vi "ts_tree_set_result.vi"(4 "results.data":string, 6 "results.txt":string, 8 "error in (no error)":errorcluster, 9 "ts.status":bool, 10 "ts.data":T1, 11 "Tree.in":refnum<vi>) -> (0 "error out":errorcluster, 3 "Tree.out":refnum<vi>)   [LabVIEW 2015]
doc: "sets the test step results for a active/parent tag"
uses:
  ts-data.ctl
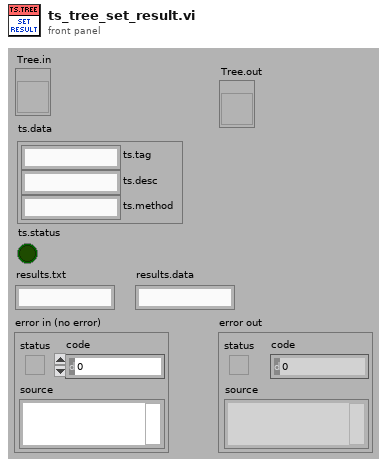
[diagram p1: front panel]
types:
  T1 = typedef "ts-data.ctl" = cluster{"ts.tag":string, "ts.desc":string, "ts.method":string}
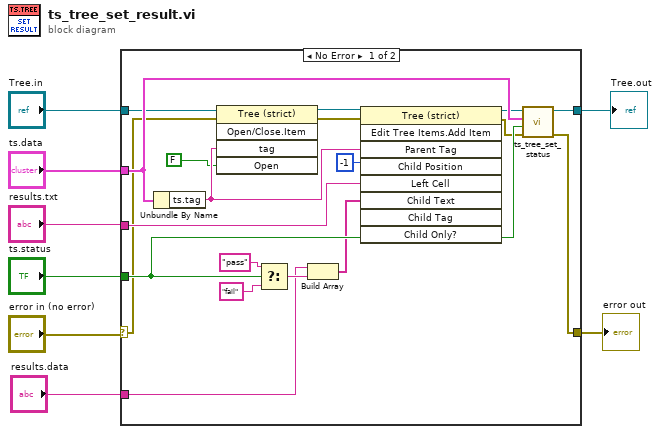
[diagram p0: block diagram]
diagram:
  n1 = case shown="No Error" "error in (no error)" {
    selector: "error in (no error)" -> [w11 w28]
    tunnel: "Tree.in" -> [w14 w29]
    tunnel: [w26 w29] -> w6
    tunnel: [w25 w28] -> w5
    tunnel: "ts.status" -> [w22 _]
    tunnel: "results.txt" -> [w24 _]
    tunnel: "ts.data" -> [w23 _]
    tunnel: "results.data" -> [w18 _]
    frame No Error {
      n2 = Unbundle By Name(w23) -> ("ts.tag"=w10:string)
      n3 = invoke class="Tree (strict)" method="Open/Close.Item"(reference=w14, error in=w11, "tag"=w10, "Open"=FALSE ("Open?")) -> (reference out=w13:refnum<vi>, error out=w12:errorcluster)  [unwired: 1 in, 3 out]
      n4 = Select(t="pass", s=w22, f="fail") -> (s? t:f=w19:string)
      n5 = Build Array(w18, w19) -> (w17:string[])
      n6 = invoke class="Tree (strict)" method="Edit Tree Items.Add Item"(reference=w13, error in=w12, "Parent Tag"=w10, "Child Position"=-1, "Left Cell"=w24, "Child Text"=w17) -> (reference out=w15:refnum<vi>, error out=w16:errorcluster)  [unwired: 3 in, 7 out]
      n7 = call "ts_tree_set_status.vi"("error in (no error)"=w16, "ts.status"=w22, "ts.data"=w23, "Tree.in"=w15) -> ("error out"=w25:errorcluster, "Tree.out"=w26:refnum<vi>)  [unwired: 6 in]
    }
    frame Error {
    }
  }
  "Tree.out" <- w6
  "error out" <- w5
